vi "make both cosine bandpass.vi"(0 "cross length":i32=128) -> (1 "Real-space cosine window":dbl[](array[numeric]), 2 "Cosine bandpass for Hilbert":dbl[](array[numeric]))   [LabVIEW 2012]
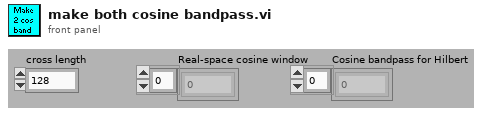
[diagram p1: front panel]
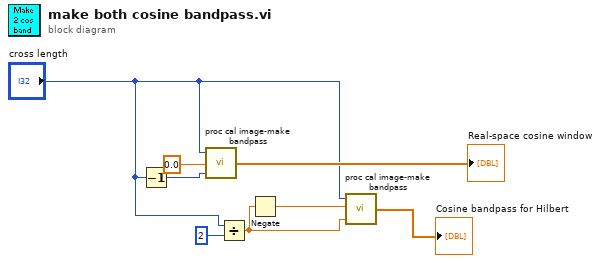
[diagram p0: block diagram]
diagram:
  n1 = Decrement(x="cross length") -> (x-1=w3:i32)
  n2 = call "proc cal image-make bandpass.vi"("HIGH bandpass\n(mode)"=w3, "LOW bandpass\n(mode)"=sgl 0.0 ("LOW bandpass\n(mode)"), "# of points (cross size)"="cross length") -> ("Cosine bandpass"=→"Real-space cosine window":sgl[])
  n3 = Divide(x="cross length", y=2) -> (x/y=w6:dbl)
  n4 = Negate(x=w6) -> (-x=w2:dbl)
  n5 = call "proc cal image-make bandpass.vi"("HIGH bandpass\n(mode)"=w6, "LOW bandpass\n(mode)"=w2, "# of points (cross size)"="cross length") -> ("Cosine bandpass"=→"Cosine bandpass for Hilbert":sgl[])
